vi "Accelerometer Remove Ofset.vi"(10 "offsets":T1, 11 "acc in":T1) -> (3 "acc out":T1)   [LabVIEW 2014]
uses:
  <vilib>/LabVIEW Universal Transcriptor/Arduino MPU6050 Library/MPU6050LibVector.ctl
  LabVIEW-Universal-Transcriptor-MPU6050-Library/Arduino MPU6050.lvlib
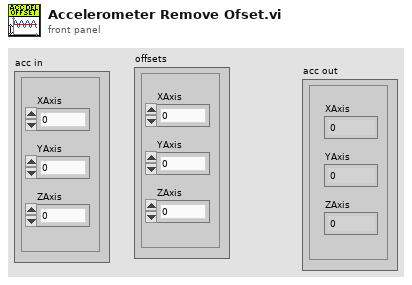
[diagram p1: front panel]
types:
  T1 = typedef "Arduino MPU6050.lvlib/MPU6050LibVector.ctl" = cluster{"XAxis":sgl, "YAxis":sgl, "ZAxis":sgl}
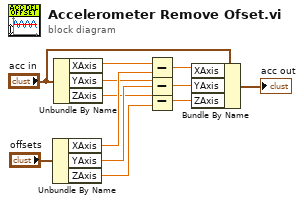
[diagram p0: block diagram]
diagram:
  n1 = Unbundle By Name("offsets") -> ("XAxis"=w9:sgl, "YAxis"=w8:sgl, "ZAxis"=w7:sgl)
  n2 = Unbundle By Name("acc in") -> ("XAxis"=w6:sgl, "YAxis"=w5:sgl, "ZAxis"=w4:sgl)
  n3 = Subtract(x=w6, y=w9) -> (x-y=w3:sgl)
  n4 = Subtract(x=w5, y=w8) -> (x-y=w2:sgl)
  n5 = Subtract(x=w4, y=w7) -> (x-y=w1:sgl)
  n6 = Bundle By Name(cluster="acc in", "XAxis"=w3, "YAxis"=w2, "ZAxis"=w1) -> (→"acc out":T1)
